vi "LABVIEW sigal processing COM port www.Electronics-Base.com.vi"() -> ()   [LabVIEW 2010]
uses:
  <vilib>/Instr/_visa.llb/VISA Configure Serial Port (Instr).vi
  <vilib>/measure/matone.llb/Extract Single Tone Information 1 Chan.vi
  <vilib>/measure/mascope.llb/Amplitude and Levels 1 chan.vi
  <vilib>/measure/NI_MAPro.lvlib
panel:
  in  "Tab Control":T1(tab)
  in  "String":string
  in  "VISA resource name":refnum<visa-resource-name>="COM4"
  in  "baud rate":u32=115200
  out "error out":errorcluster
  in  "stop":bool
  in  "COM port number of bytes":dbl=1000.0
  out "?":u8[](graph)=[92, 92, 92, 92, 92, 92, 92, 92, 92, 92, 92, 92, 92, 92, 92, 92, 92, 92, 92, 92, 92, 92, 92, 92, 92, 92, 92, 92, 92, 92, 92, 92, 92, 92, 92, 92, 92, 92, 92, 92, 92, 92, 92, 92, 92, 92, 92, 92, 92, 92, 92, 92, 92, 92, 92, 92, 92, 92, 92, 92, 92, 92, 92, 92, 92, 92, 92, 92, 92, 92, 92, 92, 92, 92, 92, 92, 92, 92, 92, 92, 92, 92, 92, 92, 92, 92, 92, 92, 92, 92, 92, 92, 92, 92, 92, 92, 92, 92, 92, 92, 92, 92, 92, 92, 92, 92, 92, 92, 92, 92, 92, 92, 92, 92, 92, 92, 92, 92, 92, 92, 92, 92, 92, 92, 92, 92, 92, 92, 92, 92, 92, 92, 92, 92, 92, 92, 92, 92, 92, 92, 92, 92, 92, 92, 92, 92, 92, 92, 92, 92, 92, 92, 92, 92, 92, 92, 92, 92, 92, 92, 92, 92, 92, 92, 92, 92, 92, 92, 92, 92, 92, 92, 92, 92, 92, 92, 92, 92, 92, 92, 92, 92, 92, 92, 92, 92, 92, 92, 0]
  out "RMS":dbl(graph)
  out "Signal amplitude":dbl(graph)
  out "Low stste level":dbl(graph)
  out "High state level":dbl(graph)
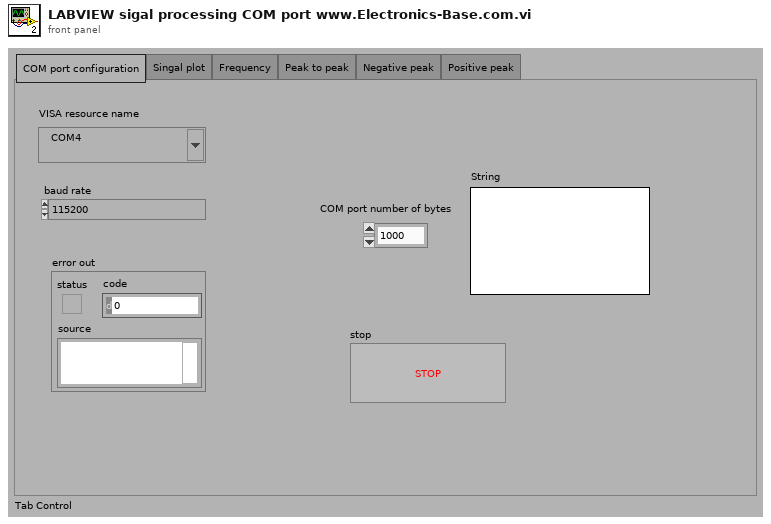
[diagram p1: front panel]
types:
  T1 = enum32{"COM port configuration", "Singal plot", "Frequency", "Peak to peak", "Negative peak", "Positive peak"}
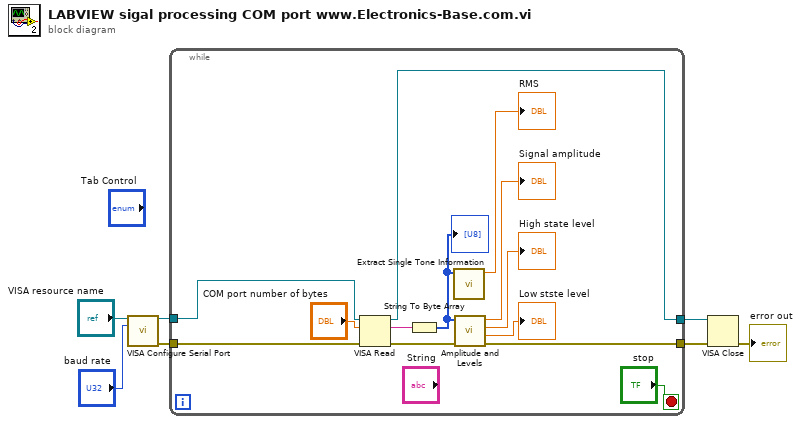
[diagram p0: block diagram]
diagram:
  n1 = call-poly "VISA Configure Serial Port"("VISA resource name"="VISA resource name", "baud rate (9600)"="baud rate") -> ("VISA resource name out"=w2:refnum<visa-resource-name>, "error out"=w1:errorcluster)  [unwired: 12 in]
  n2 = while {
    tunnel: [w19] -> w7
    tunnel: [w13] -> w6
    tunnel: w2 -> [w16]
    tunnel: w1 -> [w15]
    stop <- "stop" stop-if-true
    n3 = VISA Read(VISA resource name=w16, byte count="COM port number of bytes", error in (no error)=w15) -> (VISA resource name out=w19:refnum<visa-resource-name>, read buffer=w17:string, error out=w14:errorcluster)  [unwired: 1 out]
    n4 = String To Byte Array(string=w17) -> (unsigned byte array=w9:u8[])
    "?" <- w9
    n5 = call-poly <vilib>:"Extract Single Tone Information.vi"("time signal in"=w9) -> ("detected frequency"=→"RMS":dbl)  [unwired: 5 in, 5 out]
    n6 = call-poly <vilib>:"Amplitude and Levels.vi"("error in (no error)"=w14, "signal in"=w9) -> ("error out"=w13:errorcluster, "low state level"=→"Low stste level":dbl, "high state level"=→"High state level":dbl, "amplitude"=→"Signal amplitude":dbl)  [unwired: 6 in]
  }
  n7 = VISA Close(VISA resource name=w7, error in (no error)=w6) -> (error out=→"error out":errorcluster)
